vi "Untitled 122.vi"() -> ()   [LabVIEW 2010]
uses:
  <vilib>/NXT/Block Support/NXT_InputPort.ctl
  <vilib>/NXT/Subs/MotorOutput.ctl
  <vilib>/NXT/Dual Mode Library/Sensors/Touch_Pressed.vi
  <vilib>/NXT/Dual Mode Library/Motors/MotorOn.vi
  <vilib>/NXT/Dual Mode Library/Motors/MotorReverse.vi
  <vilib>/NXT/Dual Mode Library/Waits/Wait_Num.vi
panel:
  out "Yes / No":bool
  in  "Power (75)":i32=75
  in  "stop":bool
  in  "Time (1 sec) 2":sgl=1.0 caption="Time (1 sec)"
  in  "Time (1 sec)":sgl=1.0
  in  "Output Port (All Ports) 2":T1=3 items=["Port A", "Port B", "Port C", "All Ports"]
  in  "Output Port (All Ports)":T1=3 items=["Port A", "Port B", "Port C", "All Ports"]
  in  "Port (Port 1)":T2 items=["Port 1", "Port 2", "Port 3", "Port 4"]
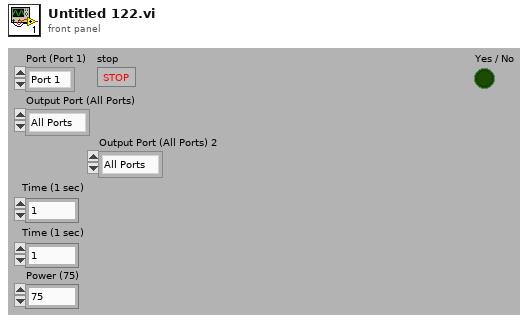
[diagram p1: front panel]
types:
  T1 = typedef "MotorOutput.ctl" = u8
  T2 = typedef "NXT_InputPort.ctl" = u8
  T3 = typedef "LVHSConnector.ctl" = cluster{"error":errorcluster, "address":string, "NXT #":i32, "Show Error":bool, "Connection":u16}
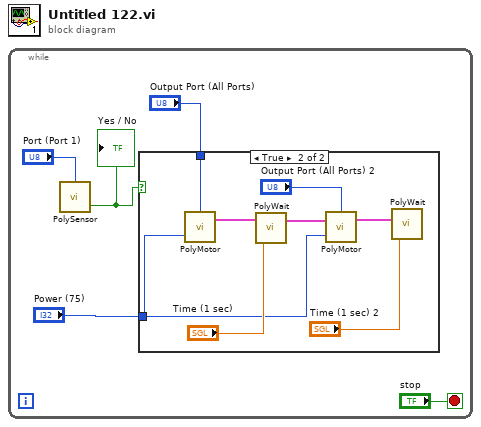
[diagram p0: block diagram]
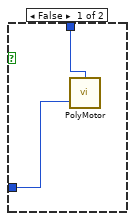
[diagram p2: hidden frame]
diagram:
  n1 = while {
    stop <- "stop" stop-if-true
    n2 = call-poly <vilib>:"PolySensor.vi"("Port (Port 1)"="Port (Port 1)") -> ("Yes / No"=w1:bool)  [unwired: 2 in, 1 out]
    "Yes / No" <- w1
    n3 = case shown="True" w1 {
      tunnel: "Output Port (All Ports)" -> [w6 w15]
      tunnel: "Power (75)" -> [w7 w8]
      frame False {
        n4 = call-poly <vilib>:"PolyMotor.vi"("Power (75)"=w7, "Output Port (All Ports)"=w6) -> ()  [unwired: 2 in, 1 out]
      }
      frame True {
        n5 = call-poly <vilib>:"PolyMotor.vi"("Power (75)"=w8, "Output Port (All Ports)"=w15) -> ("NXT"=w14:T3)  [unwired: 2 in]
        n6 = call-poly <vilib>:"PolyWait.vi"("Time (sec)"="Time (1 sec)", "NXT"=w14) -> ("NXT"=w13:T3)  [unwired: 2 in]
        n7 = call-poly <vilib>:"PolyMotor.vi"("Power (75)"=w8, "NXT"=w13, "Output Port (All Ports)"="Output Port (All Ports) 2") -> ("NXT"=w12:T3)  [unwired: 1 in]
        n8 = call-poly <vilib>:"PolyWait.vi"("Time (sec)"="Time (1 sec) 2", "NXT"=w12) -> ()  [unwired: 2 in, 1 out]
      }
    }
  }
